vi "Validate Boolean Byte Array.vi"(3 "Channel Stim Boolean Array in":bool[](array[boolean])) -> (1 "Channel Stim Boolean Array out":bool[](array[boolean]))   [LabVIEW 2019]
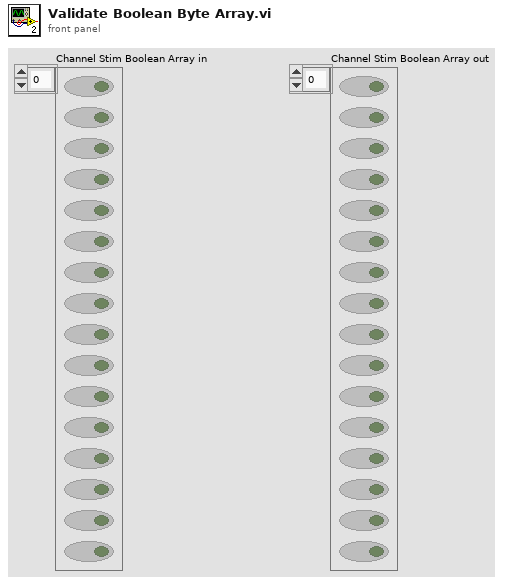
[diagram p1: front panel]
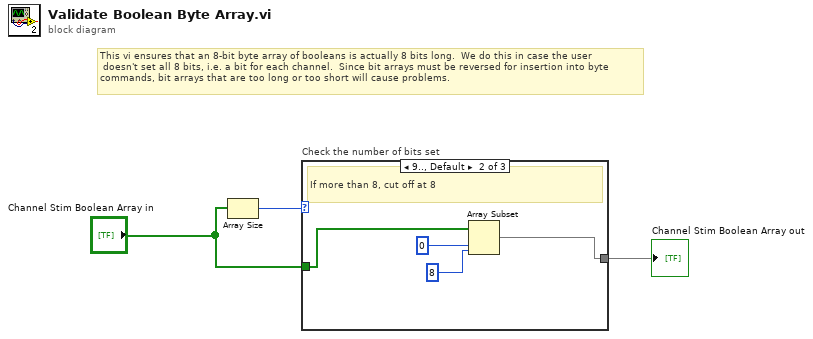
[diagram p0: block diagram]
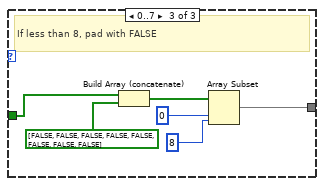
[diagram p3: hidden frame]
diagram:
  # "This vi ensures that an 8-bit byte array of booleans is actually 8 bits long.  We do this in case the user\n doesn't set all 8 bits, i.e. a bit for each channel.  Since bit arrays must be reversed for insertion into byte\ncommands, bit arrays that are too long or too short will cause problems."
  n1 = Array Size(array="Channel Stim Boolean Array in") -> (size(s)=w1:i32)
  n2 = case "Check the number of bits set" shown="9.., Default" w1 {
    tunnel: "Channel Stim Boolean Array in" -> [w4 w6 w14]
    tunnel: [w4 w5 w9] -> w3
    frame 8 {
      # "If 8, let it pass"
    }
    frame 9.., Default {
      # "If more than 8, cut off at 8"
      n3 = Array Subset(array=w6, index=0, length=8) -> (w5:bool[])
    }
    frame 0..7 {
      # "If less than 8, pad with FALSE"
      n4 = Build Array (concatenate)(w14, bool[] [FALSE, FALSE, FALSE, FALSE, FALSE, FALSE, FALSE, FALSE]) -> (w12:bool[])
      n5 = Array Subset(array=w12, index=0, length=8) -> (w9:bool[])
    }
  }
  "Channel Stim Boolean Array out" <- w3
